vi "StartSweep.vi"(10 "FIFO enabled":bool, 11 "FPGA in":refnum<queue>) -> (3 "FPGA out":refnum<queue>)   [LabVIEW 2019, in "FPGA.lvlib"]
uses:
  FPGA.lvlib
  FPGA.ctl
  Commands.ctl
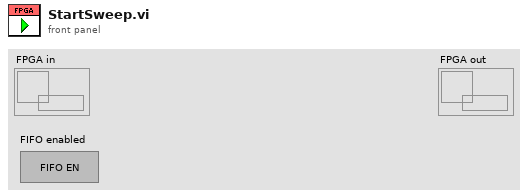
[diagram p1: front panel]
types:
  T1 = typedef "FPGA.lvlib/FPGA.ctl" = cluster{"Start freq. [Hz]":dbl, "Sweep duration [s]":dbl, "Freq. step [Hz]":dbl, "DAC Sample Rate":dbl, "ADC Sample Rate":dbl, "CMD port":u16, "DFAST port":u16, "CMD ID":refnum<k16>, "DFAST ID":refnum<k16>, "CMD error out":errorcluster, "FPGA IP":string, "DFAST error out ":errorcluster, "Stop freq. [Hz]":dbl, "Discrete sweep":bool, "Initial NCO":u32, "Difference NCO":i32, "step NCO":i64, "Final NCO":u32, "clocks for step":u32, "demodulation":bool, "NCO Phase Precision":u32, "NCO Sample Rate":dbl, "Time for step [s]":dbl, "NCO freq. resolution":dbl, "Sweep speed [Hz/s]":dbl, "Connected":bool, "Slew Rate [V/us]":dbl, "Parameters_ok":bool, "Amplitude [mVpp]":dbl, "Scale Factor":fxp<+,16,0>, "Acquiring":bool, "DAC-ADC Latency":u16, "Digital Gain":i32, "Number of steps":i32, "Averaging preferred":bool, "Filter Order":u32, "Settling":enum16{"99%", "99,9%"}, "FIFO":cluster{"Start freq. [Hz]":dbl, "Sweep duration [s]":dbl, "Freq. step [Hz]":dbl, "Stop freq. [Hz]":dbl, "Time for step [s]":dbl, "Amplitude [mVpp]":dbl, "Number of steps":i32}[]}
  T2 = typedef "FPGA.lvlib/Commands.ctl" = string
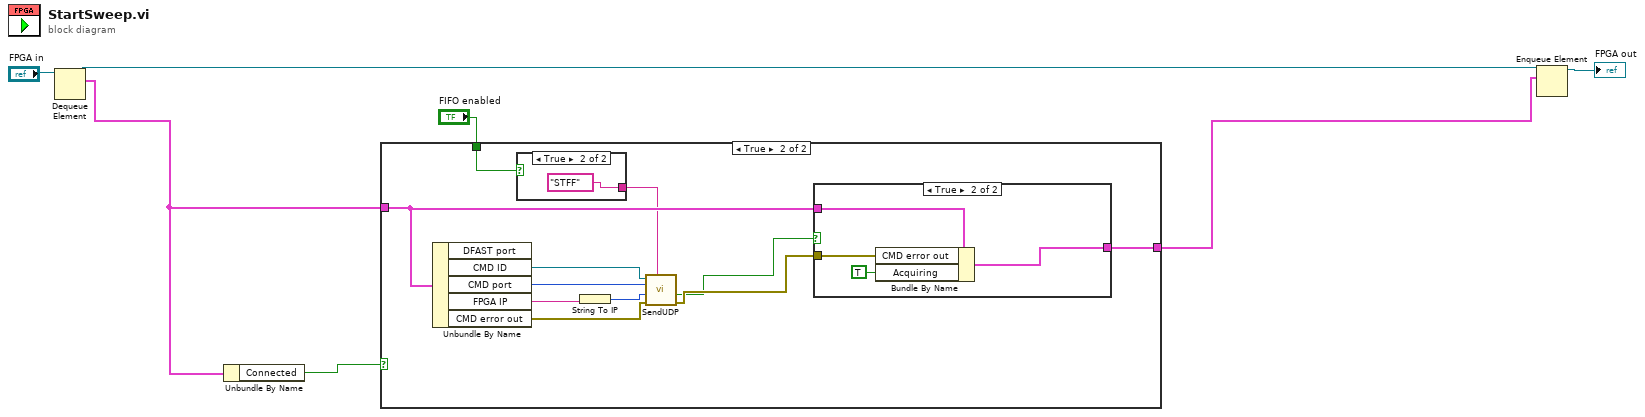
[diagram p0: block diagram]
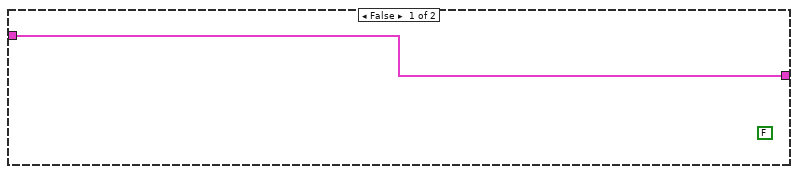
[diagram p2: hidden frame]
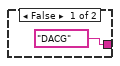
[diagram p3: hidden frame]
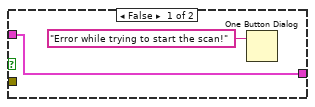
[diagram p4: hidden frame]
diagram:
  n1 = Dequeue Element(queue="FPGA in") -> (queue out=w6:refnum<queue>, element=w4:T1)  [unwired: 2 in, 2 out]
  n2 = Unbundle By Name(w4) -> ("Connected"=w2:bool)
  n3 = case shown="True" w2 {
    tunnel: w4 -> [w8 w18]
    tunnel: [w8 w17] -> w3
    tunnel: "FIFO enabled" -> [_ w9]
    frame False {
      (unwired) FALSE ("ACK")
    }
    frame True {
      n4 = Unbundle By Name(w18) -> ("CMD ID"=w16:refnum<k16>, "CMD port"=w15:u16, "FPGA IP"=w19:string, "CMD error out"=w13:errorcluster)  [unwired: 1 out]
      n5 = case shown="True" w9 {
        tunnel: [T2 "DACG" ("Combo Box") T2 "STFF" ("Combo Box")] -> w10
        frame False {
        }
        frame True {
        }
      }
      n6 = String To IP(1:w19) -> (0:w14:u32)
      n7 = call "SendUDP.vi"("data in"=w10, "error in (no error)"=w13, "address"=w14, "port or service name"=w15, "connection ID"=w16) -> ("error out"=w12:errorcluster, "ACK"=w11:bool)  [unwired: 1 in, 4 out]
      n8 = case shown="True" w11 {
        tunnel: w18 -> [w22 w27]
        tunnel: [w22 w26] -> w17
        tunnel: w12 -> [_ w25]
        frame False {
          n9 = One Button Dialog(message="Error while trying to start the scan!") -> ()  [unwired: 1 in, 1 out]
        }
        frame True {
          n10 = Bundle By Name(cluster=w27, "CMD error out"=w25, "Acquiring"=TRUE) -> (w26:T1)
        }
      }
    }
  }
  n11 = Enqueue Element(queue=w6, element=w3) -> (queue out=→"FPGA out":refnum<queue>)  [unwired: 2 in, 2 out]
